vi "Read Distance.vi"(11 "trigger/echo line":refnum<k21>="Port0/DIO0") -> (1 "timed out?":bool, 3 "distance (m)":fxp<+,32,8> format="%.27g")   [LabVIEW 2013, in "NI_Robotics_Parallax PING))) (FPGA).lvlib"]
doc: "Reads the distance in m."
uses:
  NI_Robotics_Parallax PING))) (FPGA).lvlib
  <vilib>/robotics/Utilities/FPGA Utilities/Generate Digital Pulse (uSec).vi
  <vilib>/rvi/eio/common/nirviEmuTemplateMethod_errors.vi
  <vilib>/robotics/Utilities/FPGA Utilities/Measure Digital Pulse Width (uSec).vi
  <vilib>/eio/EIOMethodNode/EIOMethodNode.xnode
  <vilib>/eio/EIONode/EIONode.xnode
  <vilib>/robotics/Utilities/FPGA Utilities/NI_Robotics_FPGA Utilities.lvlib
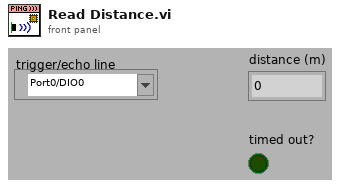
[diagram p1: front panel]
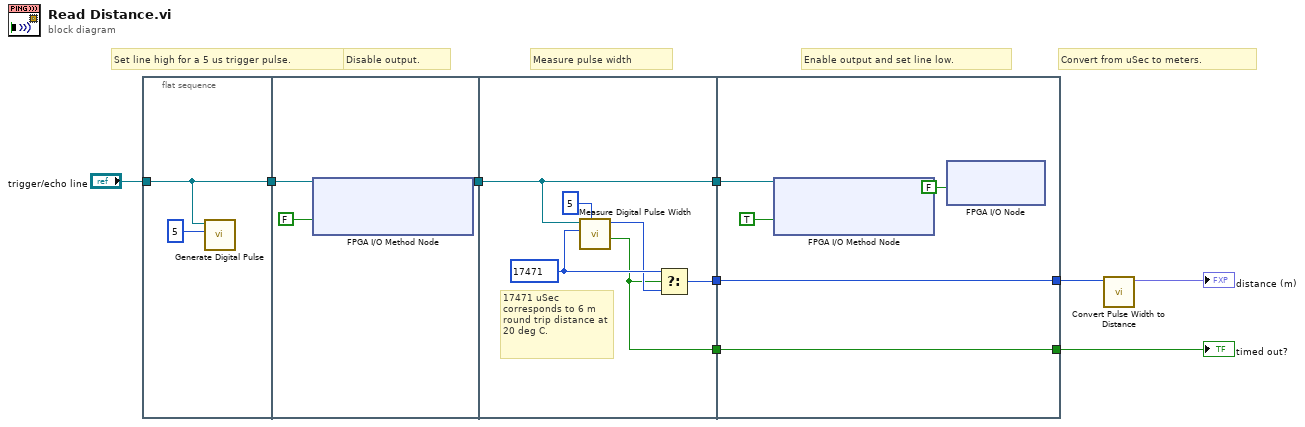
[diagram p0: block diagram]
diagram:
  # "Measure pulse width"
  # "Disable output."
  # "Convert from uSec to meters."
  # "Set line high for a 5 us trigger pulse."
  # "Enable output and set line low."
  n1 = flat-sequence {
    tunnel: [w10] -> w9
    tunnel: "trigger/echo line" -> [w10]
    tunnel: w9 -> [w13]
    tunnel: [w12] -> w8
    tunnel: w8 -> [w16]
    tunnel: [w20] -> w7
    tunnel: [w16] -> w6
    tunnel: [w17] -> w5
    tunnel: [w25] -> w3
    tunnel: [w26] -> w2
    tunnel: w7 -> [w26]
    tunnel: w6 -> [w21]
    tunnel: w5 -> [w25]
    frame #0 {
      n2 = call-poly <vilib>:"Generate Digital Pulse.vi"("pulse width (uSec)"=u32 5 ("Count(uSec)"), "FPGA digital output"=w10) -> ()  [unwired: 10 in]
    }
    frame #1 {
      n3 = xnode "FPGA I/O Method Node"("FPGA I/O In"=w13, "Enable"=FALSE) -> ("FPGA I/O Out"=w12:refnum<k21>)
    }
    frame #2 {
      w19 = 17471 ("timeout (ticks)")
      # "17471 uSec corresponds to 6 m round trip distance at 20 deg C."
      n4 = call-poly <vilib>:"Measure Digital Pulse Width.vi"("cycles to filter (0)"=u16 5, "timeout (uSec)"=w19, "FPGA digital input"=w16) -> ("timed out?"=w17:bool, "pulse width (uSec)"=w18:u32)  [unwired: 7 in]
      n5 = Select(t=w19, s=w17, f=w18) -> (s? t:f=w20:u32)
    }
    frame #3 {
      n6 = xnode "FPGA I/O Method Node"("FPGA I/O In"=w21, "Enable"=TRUE) -> ("FPGA I/O Out"=w23:refnum<k21>)
      n7 = xnode "FPGA I/O Node"("I/O Item"=FALSE, "FPGA I/O In"=w23) -> ()  [unwired: 1 out]
    }
  }
  n8 = call "Convert Pulse Width to Distance.vi"("pulse width (uSec)"=w2) -> ("distance (m)"=→"distance (m)":fxp<+,32,8>)  [unwired: 10 in]
  "timed out?" <- w3
